vi "Instanciate SessionOptions.vi"(8 "error in":errorcluster, 10 "SessionOptions in":refnum<class "SessionOptions.lvclass">) -> (0 "error out":errorcluster, 3 "Session":refnum<class "Session.lvclass">)   [LabVIEW 2015, in "LV-WinSCP.lvlib"]
uses:
  LV-WinSCP.lvlib
  Classes/SessionOptions/SessionOptions.lvclass
  Classes/Session/Session.lvclass
  C:/Program Files (x86)/WinSCP/WinSCPnet.dll
  Program Files (x86)/WinSCP/WinSCPnet.dll
  Classes/SessionOptions/SCP/SessionOptions-SCP.lvclass
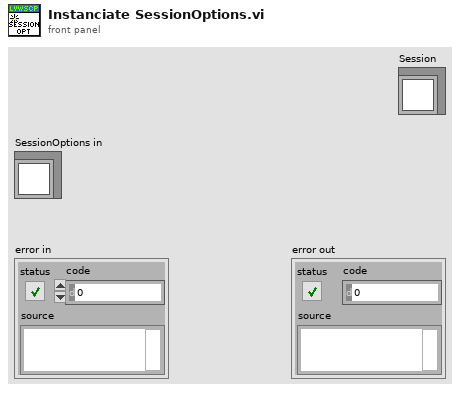
[diagram p1: front panel]
types:
  T1 = typedef "WinSCP.lvlib/SessionOptions.lvclass/Protocols--Ring.ctl" = i32
  T2 = typedef "SessionOptions-SCP.lvclass/SSHHostKeyPolicy.ctl" = i32
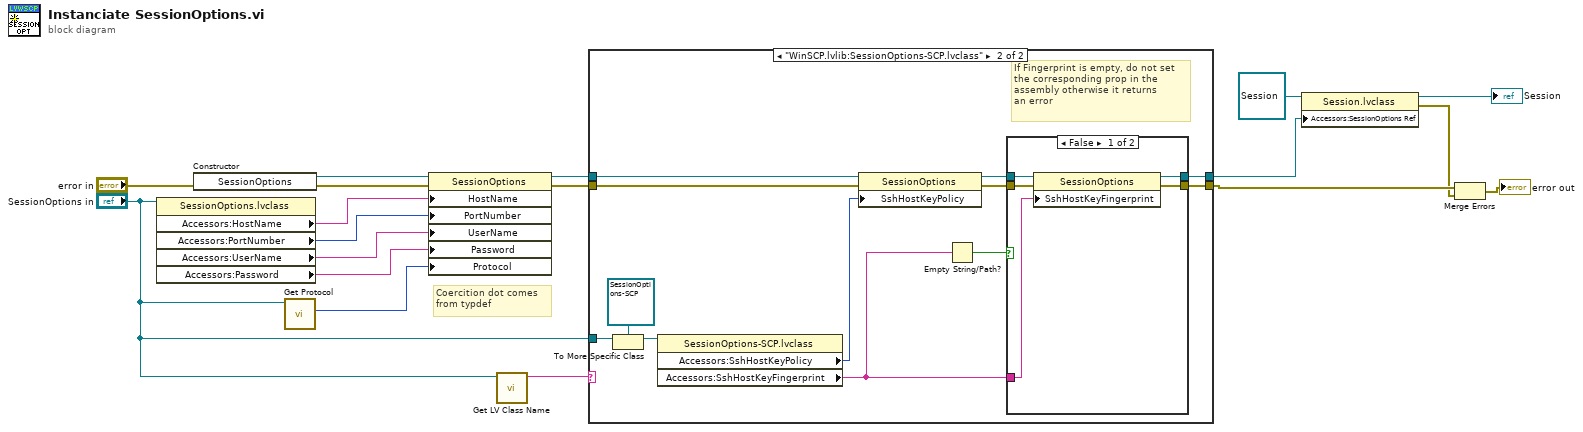
[diagram p0: block diagram]
diagram:
  # "Coercition dot comes\nfrom typdef"
  n1 = property class="SessionOptions.lvclass"(reference="SessionOptions in") -> ("Accessors:HostName"=w13:string, "Accessors:PortNumber"=w12:i32, "Accessors:UserName"=w11:string, "Accessors:Password"=w10:string)  [unwired: 1 in, 2 out]
  n2 = constructor class="SessionOptions"(error in="error in") -> (reference out=w18:refnum<k24>, error out=w15:errorcluster)  [unwired: 2 in, 1 out]
  n3 = call "Get Protocol.vi"("SessionOptions in"="SessionOptions in") -> ("Protocol"=w9:T1)  [unwired: 9 in, 1 out]
  n4 = property class="SessionOptions"(reference=w18, error in=w15, "HostName"=w13, "PortNumber"=w12, "UserName"=w11, "Password"=w10, "Protocol"=w9) -> (reference out=w16:refnum<k24>, error out=w14:errorcluster)
  n5 = call <vilib>:"Get LV Class Name.vi"("object"="SessionOptions in") -> ("class name"=w17:string)  [unwired: 9 in, 1 out]
  n6 = case shown="\"WinSCP.lvlib:SessionOptions-SCP.lvclass\"" w17 {
    tunnel: w14 -> [w19 w32]
    tunnel: w16 -> [w20 w31]
    tunnel: "SessionOptions in" -> [_ w30]
    tunnel: [w20 w24] -> w3
    tunnel: [w19 w22] -> w6
    frame "False", Default {
    }
    frame "WinSCP.lvlib:SessionOptions-SCP.lvclass" {
      # "If Fingerprint is empty, do not set\nthe corresponding prop in the\nassembly otherwise it returns \nan error"
      n7 = To More Specific Class(target class=refnum<class "SessionOptions-SCP.lvclass"> refnum ("SessionOptions-SCP.lvclass"), reference=w30) -> (specific class reference=w28:refnum<class "SessionOptions-SCP.lvclass">)  [unwired: 1 in, 1 out]
      n8 = property class="SessionOptions-SCP.lvclass"(reference=w28) -> ("Accessors:SshHostKeyPolicy"=w27:T2, "Accessors:SshHostKeyFingerprint"=w23:string)  [unwired: 1 in, 2 out]
      n9 = property class="SessionOptions"(reference=w31, error in=w32, "SshHostKeyPolicy"=w27) -> (reference out=w26:refnum<k24>, error out=w21:errorcluster)
      n10 = Empty String/Path?(string/path=w23) -> (empty?=w25:bool)
      n11 = case shown="False" w25 {
        tunnel: w26 -> [w37 w39]
        tunnel: [w35 w39] -> w24
        tunnel: w23 -> [w36 _]
        tunnel: [w34 w38] -> w22
        tunnel: w21 -> [w33 w38]
        frame False {
          n12 = property class="SessionOptions"(reference=w37, error in=w33, "SshHostKeyFingerprint"=w36) -> (reference out=w35:refnum<k24>, error out=w34:errorcluster)
        }
        frame True {
        }
      }
    }
  }
  n13 = property class="Session.lvclass"(reference=refnum<class "Session.lvclass"> refnum ("Session"), "Accessors:SessionOptions Ref"=w3) -> (reference out=→"Session":refnum<class "Session.lvclass">, error out=w1:errorcluster)  [unwired: 1 in]
  n14 = Merge Errors(w6, w1) -> (→"error out":errorcluster)
